vi "ex_GetNextChunk.vi"(8 "error in (no error)":errorcluster, 11 "file refs":T1={"file ref"=refnum, "file size (bytes:0)"=0, "read pointer (bytes:0)"=0, "chunk size (bytes:65000)"=65000}) -> (0 "error out":errorcluster, 1 "no data error":bool, 2 "chunk":string, 3 "dup file refs":T1={"file ref"=refnum, "file size (bytes:0)"=0, "read pointer (bytes:0)"=0, "chunk size (bytes:65000)"=65000}, 4 "end-of-file?":bool)   [LabVIEW 2017]
uses:
  <vilib>/express/express shared/ExFile.llb/ex_FileReference.ctl
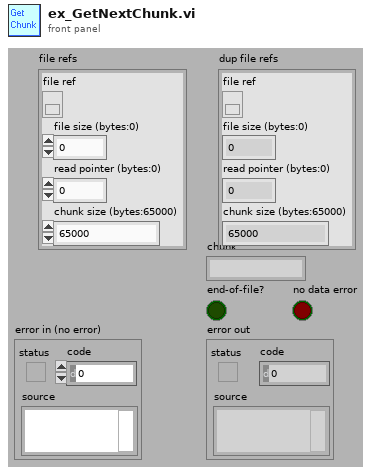
[diagram p1: front panel]
types:
  T1 = typedef "ex_FileReference.ctl" = cluster{"file ref":refnum<file>, "file size (bytes:0)":i32, "read pointer (bytes:0)":i32, "chunk size (bytes:65000)":i32}
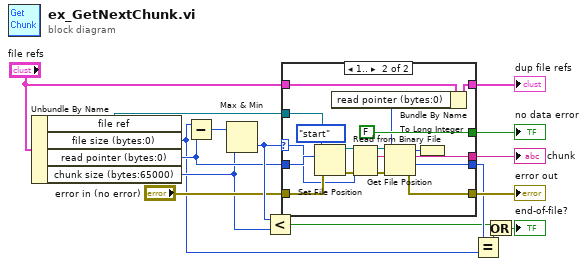
[diagram p0: block diagram]
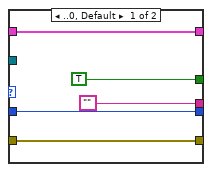
[diagram p2: hidden frame]
diagram:
  n1 = Unbundle By Name("file refs") -> ("file ref"=w10:refnum<file>, "file size (bytes:0)"=w4:i32, "read pointer (bytes:0)"=w9:i32, "chunk size (bytes:65000)"=w6:i32)
  n2 = Subtract(x=w4, y=w9) -> (x-y=w11:i32)
  n3 = Max & Min(x=w11, y=w6) -> (min(x,y)=w16:i32)  [unwired: 1 out]
  n4 = Less?(x=w16, y=w6) -> (x < y?=w2:bool)
  n5 = case shown="1.." w16 {
    selector: w16 -> [_ w28]
    tunnel: w9 -> [w17 w37]
    tunnel: "error in (no error)" -> [w21 w36]
    tunnel: w10 -> [_ w34]
    tunnel: [w21 w31] -> w13
    tunnel: ["" w33] -> w14
    tunnel: [TRUE FALSE] -> w12
    tunnel: "file refs" -> [w18 w27]
    tunnel: [w18 w29] -> w7
    tunnel: [w17 w30] -> w5
    frame ..0, Default {
    }
    frame 1.. {
      n6 = Set File Position(offset (in bytes) (0)=w37, refnum=w34, from (0:start)=enum16{"start", "end", "current"}."start" ("pos mode (0:2)"), error in=w36) -> (refnum out=w26:refnum<file>, error out=w25:errorcluster)
      n7 = Read from Binary File(8:w25, 10:w28, 11:w26) -> (0:w23:errorcluster, 2:w33:string, 3:w24:refnum<file>)  [unwired: 4 out]
      n8 = Get File Position(4:w23, 7:w24) -> (0:w31:errorcluster, 2:w22:i64)  [unwired: 1 out]
      n9 = To Long Integer(number=w22) -> (32bit integer=w30:i32)
      n10 = Bundle By Name(cluster=w27, "read pointer (bytes:0)"=w30) -> (w29:T1)
    }
  }
  "error out" <- w13
  "no data error" <- w12
  "chunk" <- w14
  "dup file refs" <- w7
  n11 = Equal?(x=w5, y=w4) -> (x = y?=w3:bool)
  n12 = Or(x=w2, y=w3) -> (x .or. y?=→"end-of-file?":bool)
